vi "Close.vi"(8 "error in (no error)":errorcluster, 11 "Instrument in":refnum<class "Instrument.lvclass">) -> (0 "error out":errorcluster, 3 "Instrument out":refnum<class "Instrument.lvclass">)   [LabVIEW 2014, in "Instrument.lvclass"]
uses:
  Instrument.lvclass
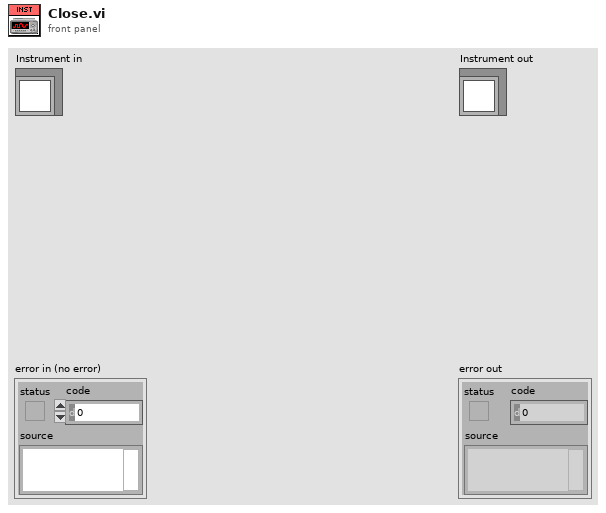
[diagram p1: front panel]
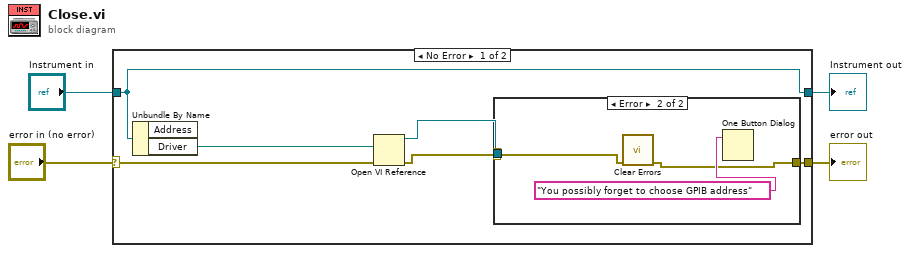
[diagram p0: block diagram]
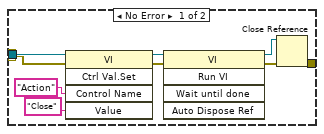
[diagram p2: hidden frame]
diagram:
  n1 = case shown="No Error" "error in (no error)" {
    selector: "error in (no error)" -> [w7 w24]
    tunnel: [w6 w24] -> w1
    tunnel: [w8 w23] -> w2
    tunnel: "Instrument in" -> [w8 w23]
    frame No Error {
      n2 = Unbundle By Name(w8) -> ("Driver"=w10:path)  [unwired: 1 out]
      n3 = Open VI Reference(vi path=w10, error in (no error)=w7) -> (vi reference=w9:refnum<vi>, error out=w5:errorcluster)  [unwired: 4 in]
      n4 = case shown="Error" w5 {
        selector: w5 -> [w11 w22]
        tunnel: w9 -> [w19 _]
        tunnel: [w12 w20] -> w6
        frame No Error {
          n5 = invoke class="VI" method="Ctrl Val.Set"(reference=w19, error in=w11, "Control Name"="Action", "Value"="Close" ("Control Name")) -> (reference out=w15:refnum<vi>, error out=w16:errorcluster)  [unwired: 1 in, 3 out]
          n6 = invoke class="VI" method="Run VI"(reference=w15, error in=w16) -> (reference out=w14:refnum<vi>, error out=w13:errorcluster)  [unwired: 3 in, 3 out]
          n7 = Close Reference(reference=w14, error in (no error)=w13) -> (error out=w12:errorcluster)
        }
        frame Error {
          n8 = call <vilib>:"Clear Errors.vi"("error in (no error)"=w22) -> ("error out"=w20:errorcluster)  [unwired: 5 in, 1 out]
          n9 = One Button Dialog(message="You possibly forget to choose GPIB address" ("error source (\" \")")) -> ()  [unwired: 1 in, 1 out]
        }
      }
    }
    frame Error {
    }
  }
  "error out" <- w1
  "Instrument out" <- w2
